vi "Add presedence for +.vi"(11 "Operators":string[](array[string])) -> (3 "Operators 2":string[](array[string]))   [LabVIEW 2018]
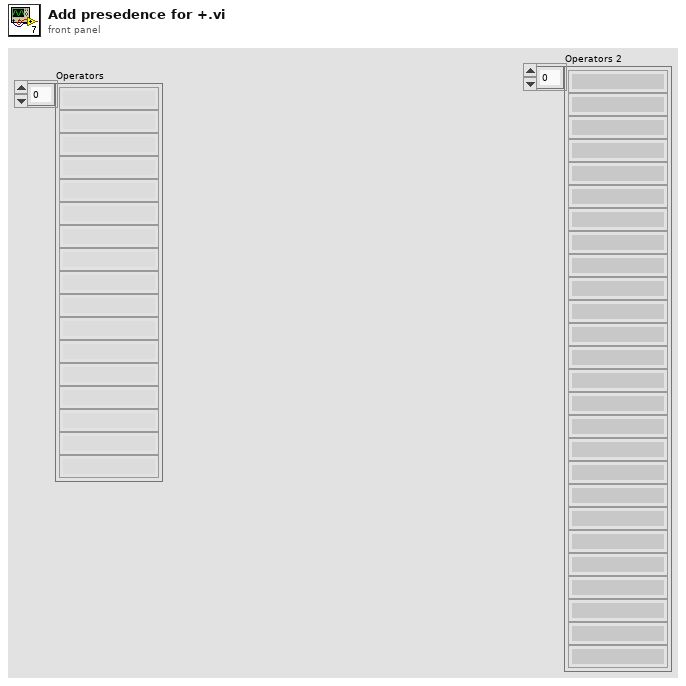
[diagram p1: front panel]
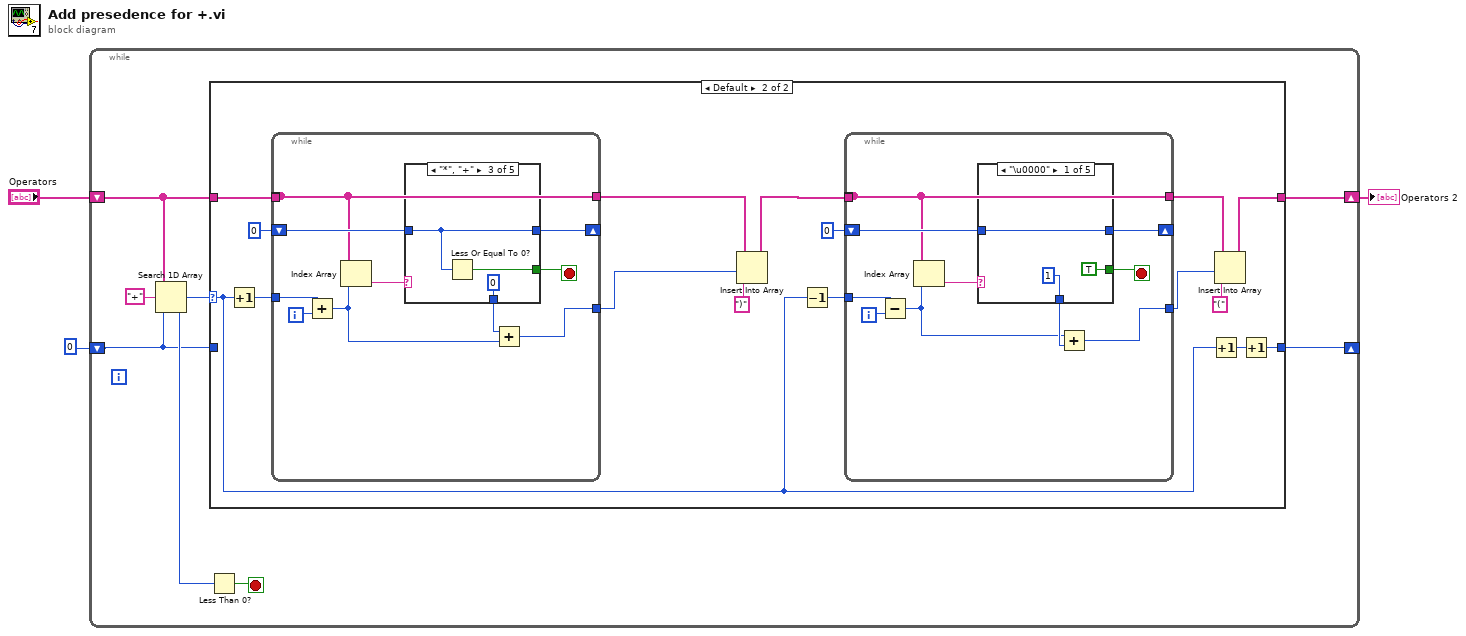
[diagram p0: block diagram]
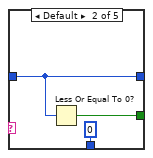
[diagram p3: hidden frame]
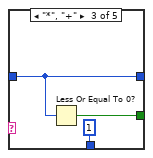
[diagram p4: hidden frame]
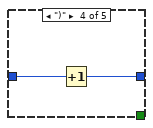
[diagram p5: hidden frame]
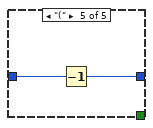
[diagram p6: hidden frame]
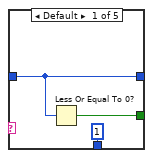
[diagram p7: hidden frame]
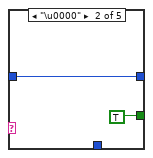
[diagram p8: hidden frame]
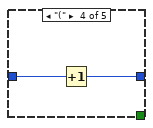
[diagram p9: hidden frame]
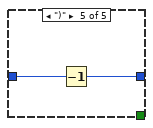
[diagram p10: hidden frame]
diagram:
  n1 = while {
    shift-right: [w6] -> w1
    shift-left: "Operators" -> [w7]
    shift-right: [w4] -> _
    shift-left: 0 -> [w5]
    stop <- w9 stop-if-true
    n2 = Search 1D Array(1D array=w7, element="+", start index (0)=w5) -> (index of element=w8:i32)
    n3 = Less Than 0?(x=w8) -> (x < 0?=w9:bool)
    n4 = case shown="Default" w8 {
      selector: w8 -> [_ w14]
      tunnel: w7 -> [w11 w28]
      tunnel: [w11 w20] -> w6
      tunnel: w5 -> [w12 _]
      tunnel: [w12 w13] -> w4
      frame -1 {
      }
      frame Default {
        n5 = Increment(x=w14) -> (x+1=w15:i32)
        n6 = while {
          tunnel: [w55] -> _
          tunnel: w28 -> [w55]
          tunnel: w15 -> [w60]
          shift-right: [w57] -> _
          shift-left: 0 -> [w58]
          tunnel: [w52] -> w17
          tunnel: [w55] -> w18
          i -> [w61]
          stop <- w56 stop-if-true
          n7 = Add(x=w60, y=w61) -> (x+y=w54:i32)
          n8 = Index Array(array=w55, index=w54) -> (element=w59:string)
          n9 = case shown="\"*\", \"+\"" w59 {
            tunnel: w58 -> [w64 w66 w69 w71 w73]
            tunnel: [w64 w66 w69 w70 w72] -> w57
            tunnel: [w63 TRUE w68 _ _] -> w56
            tunnel: [1 _ 0 _ _] -> w53
            frame Default {
              n10 = Less Or Equal To 0?(x=w64) -> (x <= 0?=w63:bool)
            }
            frame "\u0000" {
            }
            frame "*", "+" {
              n11 = Less Or Equal To 0?(x=w69) -> (x <= 0?=w68:bool)
            }
            frame "(" {
              n12 = Increment(x=w71) -> (x+1=w70:i32)
            }
            frame ")" {
              n13 = Decrement(x=w73) -> (x-1=w72:i32)
            }
          }
          n14 = Add(x=w53, y=w54) -> (x+y=w52:i32)
        }
        n15 = Insert Into Array(array=w18, index=w17, new element=")") -> (w19:string[])
        n16 = Decrement(x=w14) -> (x-1=w21:i32)
        n17 = while {
          tunnel: [w32] -> _
          tunnel: w19 -> [w32]
          tunnel: w21 -> [w37]
          shift-right: [w34] -> _
          shift-left: 0 -> [w35]
          tunnel: [w29] -> w24
          tunnel: [w32] -> w23
          i -> [w38]
          stop <- w33 stop-if-true
          n18 = Subtract(x=w37, y=w38) -> (x-y=w30:i32)
          n19 = Index Array(array=w32, index=w30) -> (element=w36:string)
          n20 = case shown="\"\"" w36 {
            tunnel: w35 -> [w41 w44 w47 w49 w51]
            tunnel: [w41 w44 w47 w48 w50] -> w34
            tunnel: [TRUE w43 w46 _ _] -> w33
            tunnel: [1 0 1 _ _] -> w31
            frame "\u0000" {
            }
            frame Default {
              n21 = Less Or Equal To 0?(x=w44) -> (x <= 0?=w43:bool)
            }
            frame "*", "+" {
              n22 = Less Or Equal To 0?(x=w47) -> (x <= 0?=w46:bool)
            }
            frame ")" {
              n23 = Increment(x=w49) -> (x+1=w48:i32)
            }
            frame "(" {
              n24 = Decrement(x=w51) -> (x-1=w50:i32)
            }
          }
          n25 = Add(x=w30, y=w31) -> (x+y=w29:i32)
        }
        n26 = Increment(x=w14) -> (x+1=w16:i32)
        n27 = Insert Into Array(array=w23, index=w24, new element="(") -> (w20:string[])
        n28 = Increment(x=w16) -> (x+1=w13:i32)
      }
    }
  }
  "Operators 2" <- w1
